vi "Measure Voltage.vi"() -> ()   [LabVIEW 2021]
doc: "Demonstrates how to use the DC Voltage Output Function to force an output voltage. This example initializes a session, configures the Output Function, Sense, Autorange, Voltage Level and Current Limit, initiates generation, waits for a specified delay, and measures the voltage and current output. This example uses Single Point source mode."
uses:
  controls/Data Holder.ctl
panel:
  out "Current Measurement 2":dbl caption="Vin SMU Current"
  out "Load SMU Current":dbl
  in  "Current Limit":dbl=0.01 format="%.3p"
  in  "Voltage Level":dbl=2.0 format="%.5p"
  in  "Load SMU":refnum<k15>="Dev1"
  in  "Load SMU Channel":string="0"
  out "Load SMU Voltage":dbl
  in  "error in":errorcluster
  out "error out":errorcluster
  out "Voltage Measurement":dbl caption="Vin SMU Voltage"
  in  "Vin SMU Channel":string="0"
  in  "Vin SMU":refnum<k15>="Dev1"
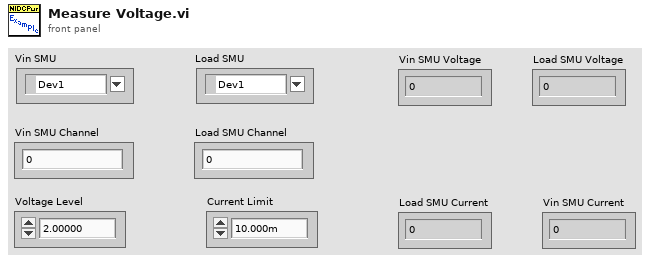
[diagram p1: front panel]
types:
  T1 = typedef "Data Holder.ctl" = cluster{"IVI Refnum in":refnum<k15>, "Vin SMU Channel":string, "Voltage Level":dbl, "Current Limit":dbl}
  T2 = typedef "Current Meas.ctl" = cluster{"Load SMU Current":dbl, "Current Measurement":dbl}
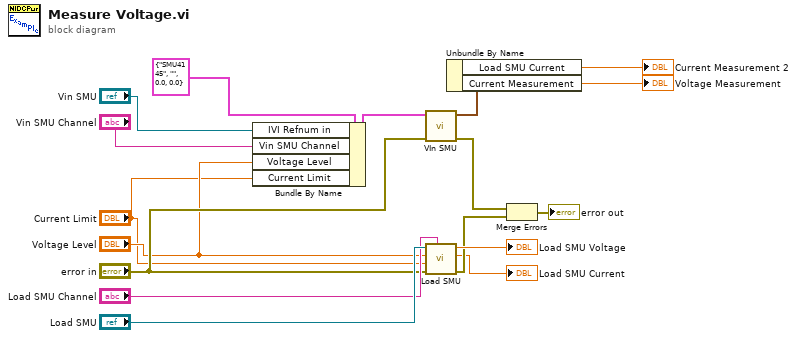
[diagram p0: block diagram]
diagram:
  n1 = Bundle By Name(cluster=T1 {"IVI Refnum in"="SMU4145", "Vin SMU Channel"="", "Voltage Level"=0.0, "Current Limit"=0.0} ("Configuration"), "IVI Refnum in"="Vin SMU", "Vin SMU Channel"="Vin SMU Channel", "Voltage Level"="Voltage Level", "Current Limit"="Current Limit") -> (w8:T1)
  n2 = call "VIn SMU.vi"("error in (no error)"="error in", "Configuration"=w8) -> ("error out"=w17:errorcluster, "Measurements"=w3:T2)  [unwired: 8 in]
  n3 = call "Load SMU.vi"("Load SMU Channel"="Load SMU Channel", "error in (no error)"="error in", "Current Limit"="Current Limit", "Voltage Level"="Voltage Level", "IVI Refnum in"="Load SMU") -> ("error out"=w13:errorcluster, "Numeric"=→"Load SMU Current":dbl, "Numeric 2"=→"Load SMU Voltage":dbl)  [unwired: 4 in]
  n4 = Unbundle By Name(w3) -> ("Load SMU Current"=→"Current Measurement 2":dbl, "Current Measurement"=→"Voltage Measurement":dbl)
  n5 = Merge Errors(w17, w13) -> (→"error out":errorcluster)
